vi "Receive Message.vi"(6 "priority":i32, 10 "Sequencer in":refnum<class "Sequencer.lvclass">, 11 "Message in":refnum<class "Message.lvclass">) -> (0 "error out":errorcluster, 2 "Actor out":refnum<class "Actor.lvclass">)   [LabVIEW 2020, in "Sequencer.lvlib" / "Sequencer.lvclass"]
doc: "Auto forward all messages to the Sequencer Core. Only exceptions are messages from the Sequencer Msg hierarchy."
uses:
  Sequencer.lvclass
  PPL/HDH.Actor Framework.Core.Actor.lvlibp/1abvi3w/vi.lib/ActorFramework/Message/Message.lvclass
  PPL/HDH.Actor Framework.Core.Actor.lvlibp/1abvi3w/vi.lib/ActorFramework/Actor/Actor.lvclass
  C:/Current projects/WS/PPL/HDH.Actor Framework.Core.Actor.lvlibp/1abvi3w/vi.lib/ActorFramework/Actor/Actor.lvclass
  PPL/HDH.Actor Framework.Core.Actor.lvlibp/1abvi3w/vi.lib/ActorFramework/Stop Msg/Stop Msg.lvclass
  Sequencer Messages/Sequencer Msg/Sequencer Msg.lvclass
  Sequencer Messages/Sequencer Msg/Sequencer Msg.lvclass/Sequencer Msg.ctl
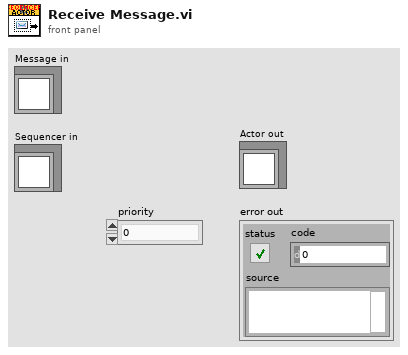
[diagram p1: front panel]
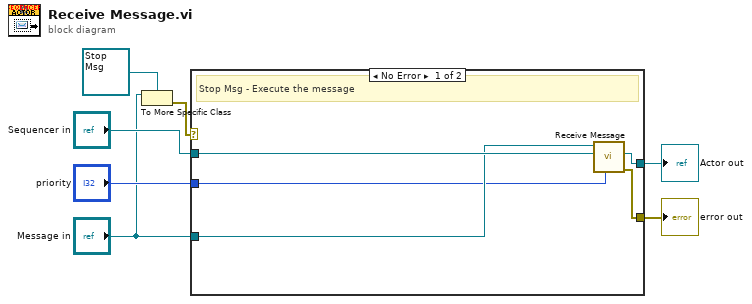
[diagram p0: block diagram]
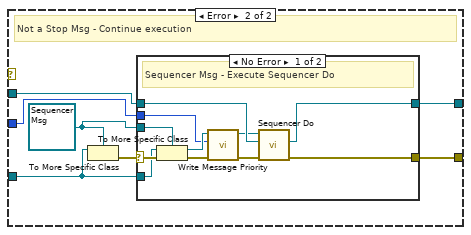
[diagram p2: hidden frame]
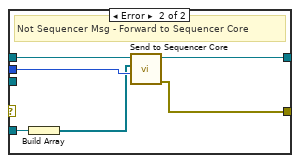
[diagram p3: hidden frame]
diagram:
  n1 = To More Specific Class(target class=refnum<class "Stop Msg.lvclass"> refnum ("Actor Framework:Stop Msg"), reference="Message in") -> (error out=w1:errorcluster)  [unwired: 1 in, 1 out]
  n2 = case shown="No Error" w1 {
    tunnel: [w10 w19] -> w7
    tunnel: [w11 w18] -> w6
    tunnel: "priority" -> [w8 w17]
    tunnel: "Sequencer in" -> [w12 w16]
    tunnel: "Message in" -> [w9 w13]
    frame No Error {
      # "Stop Msg - Execute the message"
      n3 = call-parent "Receive Message.vi"("priority"=w8, "Actor in"=w12, "Message in"=w9) -> ("error out"=w10:errorcluster, "Actor out"=w11:refnum<class "Actor.lvclass">)  [unwired: 7 in]
    }
    frame Error {
      w14 = refnum<class "Sequencer Msg.lvclass"> refnum ("Sequencer.lvlib:Sequencer Msg.lvclass")
      # "Not a Stop Msg - Continue execution"
      n4 = To More Specific Class(target class=w14, reference=w13) -> (error out=w15:errorcluster)  [unwired: 1 in, 1 out]
      n5 = case shown="No Error" w15 {
        selector: w15 -> [w30 _]
        tunnel: [w27 w33] -> w19
        tunnel: [w25 w35] -> w18
        tunnel: w17 -> [w20 w34]
        tunnel: w16 -> [w26 w36]
        tunnel: w13 -> [w29 w32]
        tunnel: w14 -> [w28 _]
        frame No Error {
          # "Sequencer Msg - Execute Sequencer Do"
          n6 = To More Specific Class(target class=w28, reference=w29, error in=w30) -> (specific class reference=w24:refnum<class "Sequencer Msg.lvclass">, error out=w22:errorcluster)
          n7 = call "Write Message Priority.vi"("error in (no error)"=w22, "Priority"=w20, "Sequencer Msg in"=w24) -> ("error out"=w21:errorcluster, "Sequencer Msg out"=w23:refnum<class "Sequencer Msg.lvclass">)  [unwired: 7 in]
          n8 = call-dynamic "Sequencer Do.vi"("error in (no error)"=w21, "Sequencer in"=w26, "Sequencer Msg"=w23) -> ("error out"=w27:errorcluster, "Sequencer out"=w25:refnum<class "Sequencer.lvclass">)  [unwired: 7 in]
        }
        frame Error {
          # "Not Sequencer Msg - Forward to Sequencer Core"
          n9 = Build Array(w32) -> (w31:refnum<class "Message.lvclass">[])
          n10 = call "Send to Sequencer Core.vi"("Message Priority"=w34, "Message Array"=w31, "Sequencer in"=w36) -> ("error out"=w33:errorcluster, "Sequencer out"=w35:refnum<class "Sequencer.lvclass">)  [unwired: 7 in]
        }
      }
    }
  }
  "error out" <- w7
  "Actor out" <- w6
